vi "Volts_to_mag_field__(SubVI).vi"(1 "делитель":dbl, 4 "U":i32, 13 "k":dbl, 14 "zero lvl":dbl) -> (9 "s? color":u32, 10 "Vin < 0?":bool, 21 "meas_voltage":dbl, 24 "B":dbl)   [LabVIEW 2015]
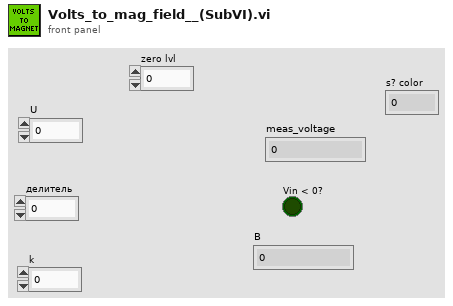
[diagram p1: front panel]
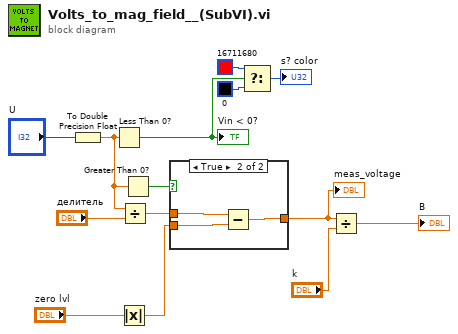
[diagram p0: block diagram]
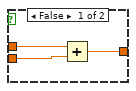
[diagram p2: hidden frame]
diagram:
  n1 = To Double Precision Float(number="U") -> (double precision float=w3:dbl)
  n2 = Less Than 0?(x=w3) -> (x < 0?=w12:bool)
  "Vin < 0?" <- w12
  n3 = Absolute Value(x="zero lvl") -> (abs(x)=w1:dbl)
  n4 = Divide(x=w3, y="делитель") -> (x/y=w5:dbl)
  n5 = Greater Than 0?(x=w3) -> (x > 0?=w7:bool)
  n6 = case shown="True" w7 {
    tunnel: w1 -> [w15 w18]
    tunnel: w5 -> [w16 w19]
    tunnel: [w17 w20] -> w4
    frame False {
      n7 = Add(x=w16, y=w15) -> (x+y=w17:dbl)
    }
    frame True {
      n8 = Subtract(x=w19, y=w18) -> (x-y=w20:dbl)
    }
  }
  "meas_voltage" <- w4
  n9 = Select(t=u32 16711680, s=w12, f=u32 0) -> (s? t:f=→"s? color":u32)
  n10 = Divide(x=w4, y="k") -> (x/y=→"B":dbl)
